vi "Measurement Item Setup.vi"(8 "error in (no error)":errorcluster, 9 "Element (0: All)":u16(ring)=1 items=["All", "Element 1", "Element 2", "Element 3", "Sigma"], 10 "i-j":i32, 11 "VISA Refnum in":refnum<visa-resource-name>) -> (0 "error out":errorcluster, 1 "Actual output":u16[][](array[numeric]), 2 "i-j 2":i32, 3 "VISA Refnum out":refnum<visa-resource-name>, 4 "position":i32[](array[numeric]))   [LabVIEW 2013, in "Universal Power Meter.lvlib" / "Yokogawa WT500.lvlib" / "Yokogawa WT500.lvclass"]
uses:
  Yokogawa WT500.lvclass
panel:
  out "Function":u16[](array[ring])=[1, 6, 11, 16, 25, 28, 55, 56] items=["None", "Urms", "Umn", "Udc", "Urmn", "Uac", "Irms", "Imn", "Idc", "Irmn", "Iac", "P", "S", "Q", "Lambda", "Phi", "Freq U", "Freq I", "U +peak", "U -peak", "I +peak", "I -peak", "Cf U", "Cf I", "Time", "Wp", "Wp+", "Wp-", "q", "q+", "q-", "WS", "WQ", "Eta 1", "Eta 2", "F1", "F2", "F3", "F4", "F5", "F6", "F7", "F8", "U(k)", "I(k)", "P(k)", "S(k)", "Q(k)", "Lambda(k)", "Phi(k)", "Phi U(k)", "Phi I(k)", "Uhdf(k)", "Ihdf(k)", "Phdf(k)", "Uthd", "Ithd", "Pthd", "Phi Ui-Uj", "Phi Ui-Uk", "Phi Ui-Ii", "Phi Ui-Ij", "Phi Ui-Ik", "Delta 1", "Delta 2", "Delta 3", "Delta 4"]
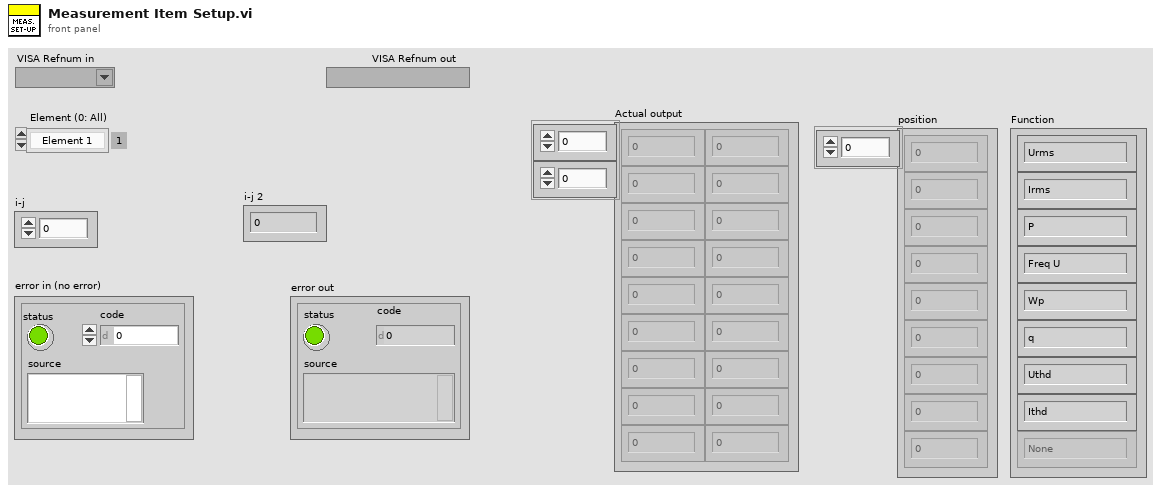
[diagram p1: front panel]
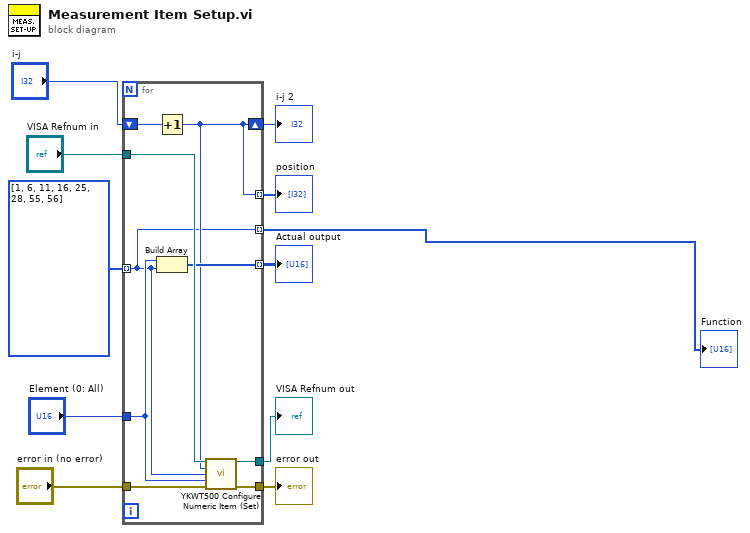
[diagram p0: block diagram]
diagram:
  w9 = u16[] [1, 6, 11, 16, 25, 28, 55, 56] items=["None", "Urms", "Umn", "Udc", "Urmn", "Uac", "Irms", "Imn", "Idc", "Irmn", "Iac", "P", "S", "Q", "Lambda", "Phi", "Freq U", "Freq I", "U +peak", "U -peak", "I +peak", "I -peak", "Cf U", "Cf I", "Time", "Wp", "Wp+", "Wp-", "q", "q+", "q-", "WS", "WQ", "Eta 1", "Eta 2", "F1", "F2", "F3", "F4", "F5", "F6", "F7", "F8", "U(k)", "I(k)", "P(k)", "S(k)", "Q(k)", "Lambda(k)", "Phi(k)", "Phi U(k)", "Phi I(k)", "Uhdf(k)", "Ihdf(k)", "Phdf(k)", "Uthd", "Ithd", "Pthd", "Phi Ui-Uj", "Phi Ui-Uk", "Phi Ui-Ii", "Phi Ui-Ij", "Phi Ui-Ik", "Delta 1", "Delta 2", "Delta 3", "Delta 4"] ("Function")
  n1 = for {
    tunnel: "VISA Refnum in" -> [w20]
    tunnel: [w19] -> w11
    tunnel: w9 -> [w12] mode=indexing
    tunnel: [w18] -> w7
    tunnel: "Element (0: All)" -> [w16]
    tunnel: "error in (no error)" -> [w17]
    tunnel: [w15] -> w5 mode=indexing
    shift-right: [w13] -> w3
    shift-left: "i-j" -> [w14]
    tunnel: [w13] -> w2 mode=indexing
    tunnel: [w12] -> w1 mode=indexing
    n2 = Increment(x=w14) -> (x+1=w13:i32)
    n3 = Build Array(w16, w12) -> (w15:u16[])
    n4 = call <instrlib>:"YKWT500 Configure Numeric Item (Set).vi"("VISA resource name"=w20, "Numeric Item Number (1)"=w13, "Numeric Function (0: None)"=w12, "Element (1: Element 1)"=w16, "error in (no error)"=w17) -> ("VISA resource name out"=w19:refnum<visa-resource-name>, "error out"=w18:errorcluster)  [unwired: 9 in]
  }
  "VISA Refnum out" <- w11
  "error out" <- w7
  "Actual output" <- w5
  "i-j 2" <- w3
  "position" <- w2
  "Function" <- w1
